vi "hold variable.vi"() -> ()   [LabVIEW 2022 SP3, in "超标留样集成.lvlib" / "DR803M4.lvlib"]
uses:
  DR803M4.lvlib
panel:
  out "通讯":bool
  in  "Slave ID":u8=1
  in  "VISA Resource":refnum<visa-resource-name>="COM9"
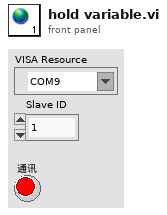
[diagram p1: front panel]
diagram:
